vi "tank-overflow-detector.vi"() -> ()   [LabVIEW 2025]
panel:
  in  "Knob":dbl(knob) scale=0.0..10.0
  out "< 2":bool
  out "> 8":bool
  out "Tank":dbl(slide) scale=0.0..10.0
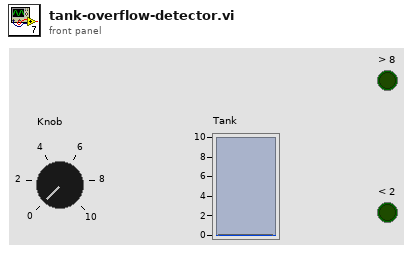
[diagram p1: front panel]
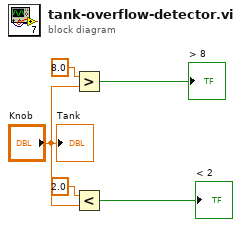
[diagram p0: block diagram]
diagram:
  n1 = Greater?(x=8.0, y="Knob") -> (0:→"> 8":bool)
  n2 = Less?(x=2.0, y="Knob") -> (x < y?=→"< 2":bool)
  "Tank" <- "Knob"
